vi "student_transmitter.vi"() -> ()   [LabVIEW 2021]
uses:
  <vilib>/sound2/lvsound2.llb/Sound Data Format.ctl
  <vilib>/addons/Modulation/Analog/support/mod_Set Error Source.vi
  <vilib>/sound2/lvsound2.llb/Sound File Info (path).vi
  <vilib>/addons/Modulation/Digital/Support/Common/Validators/mod_Generate Filter Coefficients Validate.vi
  <vilib>/addons/Modulation/Digital/General/subVIs/mod_Generate Filter Coefficients.vi
  <vilib>/addons/Modulation/Digital/General/MT Generate PSK System Parameters(M).vi
  <instrlib>/niUSRP/niUSRP Write Tx Data (CDB).vi
  <vilib>/addons/Modulation/niDMT.lvlib
panel:
  out "data":waveform(dbl)[](array[waveform])
  in  "samples per symbol (16)":i32=16
  in  "differential PSK":enum16{"disable", "enable"}(ring)
  out "sound format":T1={"sample rate (S/s)"=22050.0, "number of channels"=2, "bits per sample"=16}
  in  "matched samples per symbol (16)":i32=16
  in  "Path input":path
  out "Constellation Graph":T2(graph)
  in  "pulse shaping samples per symbol (16)":i32=16
  in  "pulse shaping filter (none)":T3(ring)
  out "error out":errorcluster
  in  "reset? (T)":bool=TRUE
  in  "active antenna":string
  in  "gain":dbl format="%#_6f"
  in  "carrier frequency":dbl=100000.0 format="%#_6p"
  in  "IQ rate":dbl=100000.0 format="%#_6p"
  in  "error in (no error)":errorcluster
  in  "USRP IP Address":refnum<k15>
  in  "stop":bool
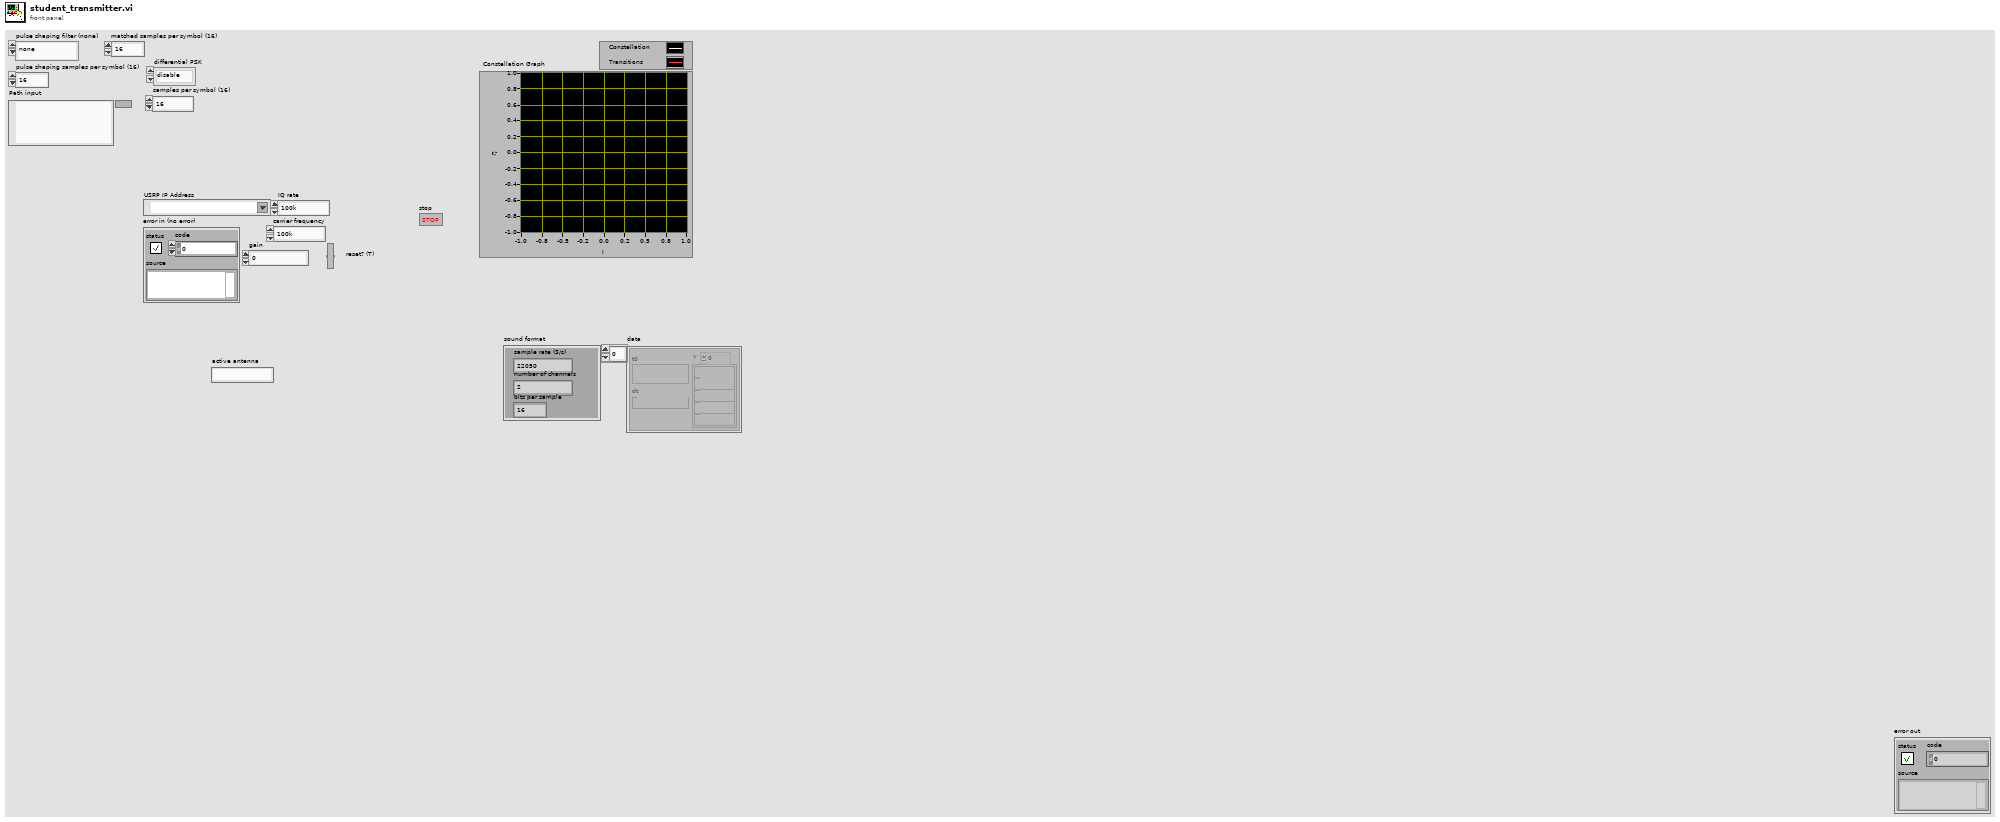
[diagram p1: front panel]
types:
  T1 = typedef "Sound Data Format.ctl" = cluster{"sample rate (S/s)":dbl, "number of channels":i32, "bits per sample":i32}
  T2 = cluster{"Decimated Array":dbl[], "Decimated Array":dbl[]}[]
  T3 = enum16{"none", "Raised Cosine", "Root Raised Cos", "Gaussian"}
  T4 = enum16{"FSK", "PSK", "QAM", "MSK", "PAM", "ASK", "CPM"}
  T5 = cluster{"samples per symbol (16)":i32, "symbol map":cdb[], "differential PSK":enum16{"disable", "enable"}, "PSK type":u16}
  T6 = typedef "niAMT.lvlib/Complex Data Waveform.ctl" = cluster{"t0":dbl, "dt":dbl, "Y":cdb[]}
  T7 = cluster{"constellation":dbl[], "oversampled data":dbl[]}[]
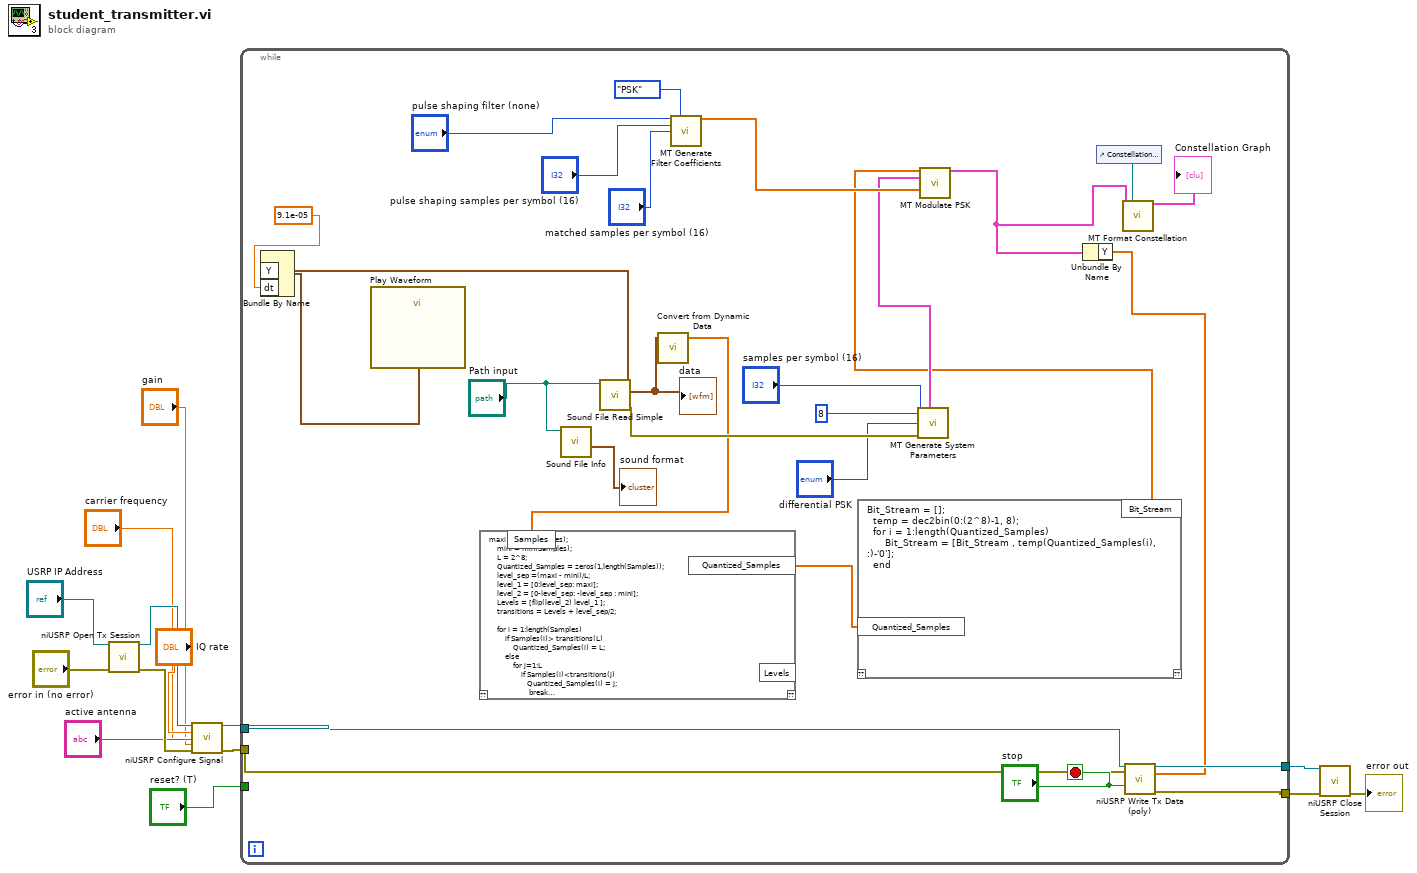
[diagram p0: block diagram]
diagram:
  n1 = call <instrlib>:"niUSRP Open Tx Session.vi"("device names"="USRP IP Address", "error in (no error)"="error in (no error)") -> ("session handle out"=w14:refnum<k15>, "error out"=w13:errorcluster)  [unwired: 12 in]
  n2 = call <instrlib>:"niUSRP Configure Signal.vi"("session handle"=w14, "IQ rate"="IQ rate", "carrier frequency"="carrier frequency", "gain"="gain", "error in (no error)"=w13, "active antenna"="active antenna") -> ("session handle out"=w1:refnum<k15>, "error out"=w5:errorcluster)  [unwired: 5 in, 3 out]
  n3 = while {
    tunnel: [w41] -> w2
    tunnel: [w40] -> w3
    tunnel: w5 -> [w37]
    tunnel: "reset? (T)" -> [_]
    tunnel: w1 -> [w38]
    stop <- "stop" stop-if-true
    n4 = call-poly <vilib>:"Sound File Info.vi"("path"="Path input") -> ("sound format"=→"sound format":T1)  [unwired: 7 in, 3 out]
    n5 = call <vilib>:"Sound File Read Simple.vi"("path"="Path input") -> ("error out"=w27:errorcluster, "data"=w15:waveform(dbl)[])  [unwired: 7 in, 2 out]
    "data" <- w15
    n6 = Bundle By Name("Y"=w15, "dt"=9.1e-05) -> (w17:waveform(dbl))  [unwired: 1 in]
    n7 = call "Play Waveform"("Data"=w17) -> ()  [unwired: 18 in, 1 out]
    n8 = call "Convert from Dynamic Data"("Dynamic Data Type"=w15) -> ("Array"=w20:dbl[])  [unwired: 3 in]
    n9 = script code="maxi = max(Samples);\n    mini = min(Samples);\n    L = 2^8;\n    Quantized_Samples = zeros(1,length(Samples));\n    level_sep =(maxi - mini)/L; \n    level_1 = [0:level_sep: maxi];\n    level_2 = [0-level_sep: -level_sep : mini];\n    Levels = [flip(level_2) level_1 ];\n    transitions = Levels + level_sep/2;\n    \n    for i = 1:length(Samples)\n        if Samples(i)> transitions(L)\n            Quantized_Samples(i) = L;\n        else\n            for j=1:L\n                if Samples(i)<transitions(j)\n                   Quantized_Samples(i) = j;\n                    break\n                end\n            end\n        end\n    end"("Samples"=w20) -> ("Quantized_Samples"=w22:dbl[])  [unwired: 1 in, 2 out]
    n10 = call <vilib>:"MT Generate Filter Coefficients.vi"("pulse shaping filter (none)"="pulse shaping filter (none)", "modulation type"=T4."PSK", "pulse shaping samples per symbol (16)"="pulse shaping samples per symbol (16)", "matched samples per symbol (16)"="matched samples per symbol (16)") -> ("pulse shaping filter coefficients"=w32:dbl[])  [unwired: 9 in, 2 out]
    n11 = script code="Bit_Stream = [];\n  temp = dec2bin(0:(2^8)-1, 8);  \n  for i = 1:length(Quantized_Samples)\n      Bit_Stream = [Bit_Stream , temp(Quantized_Samples(i), :)-'0'];\n  end"("Quantized_Samples"=w22) -> ("Bit_Stream"=w21:dbl[])  [unwired: 1 in, 1 out]
    n12 = call-poly <vilib>:"MT Generate System Parameters.vi"("samples per symbol (16)"="samples per symbol (16)", "M-PSK (4)"=8, "differential PSK"="differential PSK", "error in (no error)"=w27) -> ("PSK system parameters"=w23:T5)  [unwired: 9 in, 2 out]
    n13 = call <vilib>:"MT Modulate PSK.vi"("input bit stream"=w21, "PSK system parameters"=w23, "pulse shaping filter coefficients"=w32) -> ("output complex waveform"=w19:T6)  [unwired: 10 in, 2 out]
    n14 = Unbundle By Name(w19) -> ("Y"=w18:cdb[])
    n15 = control-ref of="Constellation Graph"() -> (w34:refnum<vi>)
    n16 = call <vilib>:"MT Format Constellation.vi"("waveform"=w19, "constellation reference"=w34) -> ("constellation graph"=→"Constellation Graph":T7)  [unwired: 3 in, 10 out]
    n17 = call-poly <instrlib>:"niUSRP Write Tx Data (poly).vi"("session handle"=w38, "data"=w18, "end of data?"="stop", "error in (no error)"=w37) -> ("session handle out"=w40:refnum<k15>, "error out"=w41:errorcluster)  [unwired: 10 in]
  }
  n18 = call <instrlib>:"niUSRP Close Session.vi"("session handle"=w3, "error in (no error)"=w2) -> ("error out"=→"error out":errorcluster)  [unwired: 13 in]
